vi "Write_output_file.vi"(0 "Output filename":path, 1 "Header":string, 2 "Template Filename":path, 5 "Channel Names":string[](array[string]), 7 "Data":string[][](array[string]), 9 "Desired Columns":i32[](array[numeric])=[0, 1, 2, 3, 4, 5, 6, 7, 8, 9, 10, 11, 12, 13, 14, 15, 16, 17, 18, 19, 20, 21, 22, 23, 24, 25, 26, 27, 28, 29, 30, 31, 32, 33, 34, 35, 36, 37, 38, 39, 40, 41, 42, 43, 44, 45, 46, 47, 48, 49, 50, 51, 52, 53, 54, 55, 56, 57, 58, 59, 60, 61, 62, 63, 64, 65, 66, 67, 68, 69, 70, 71, 72, 73, 74, 75, 76, 77, 78, 79, 80, 81, 82, 83, 84, 85, 86, 87, 88, 89, 90, 91, 92, 93, 94, 95, 96, 97, 98, 99, 100, 101, 102, 103, 104, 105, 106, 107, 108, 109, 110, 111, 112, 113, 114, 115, 116, 117, 118, 119, 120, 121, 122, 123, 124, 125, 126, 127, 128, 129, 130, 131, 132, 133, 134, 135, 136, 137, 138, 139, 140, 141, 142, 143, 144, 145, 146, 147, 148, 149, 150, 151, 152, 153, 154, 155, 156, 157, 158, 159, 160, 161, 162, 163, 164, 165, 166, 167, 168, 169, 170, 171, 172, 173, 174, 175, 176, 177, 178, 179, 180, 181, 182, 183, 184, 185, 186, 187, 188, 189, 190, 191, 192, 193, 194, 195, 196, 197, 198, 199, 200, 201, 202, 203, 204, 205, 206, 207, 208, 209, 210, 211, 212, 213, 214, 215, 216, 217, 218, 219, 220, 221, 222, 223, 224, 225, 226, 227, 228, 229, 230, 231, 232, 233, 234], 11 "Simple Save?":bool, 12 "Save Plotted rows only?":bool, 13 "Summarise mode":T2(ring), 14 "Grouping info":T3[](array[typedef]), 15 "Channels to Tabulate in header":i32[](listbox)) -> (4 "Output filename Out":path)   [LabVIEW 2020]
uses:
  Controls/Group_Binning.ctl
  Results_plotter_Global.vi
panel:
  out "Which Button?":T1(ring)=enum."Center Button"
  out "Table Values":string[][](array[string])
  out "Table Names":string[](array[string])
  out "Table":string
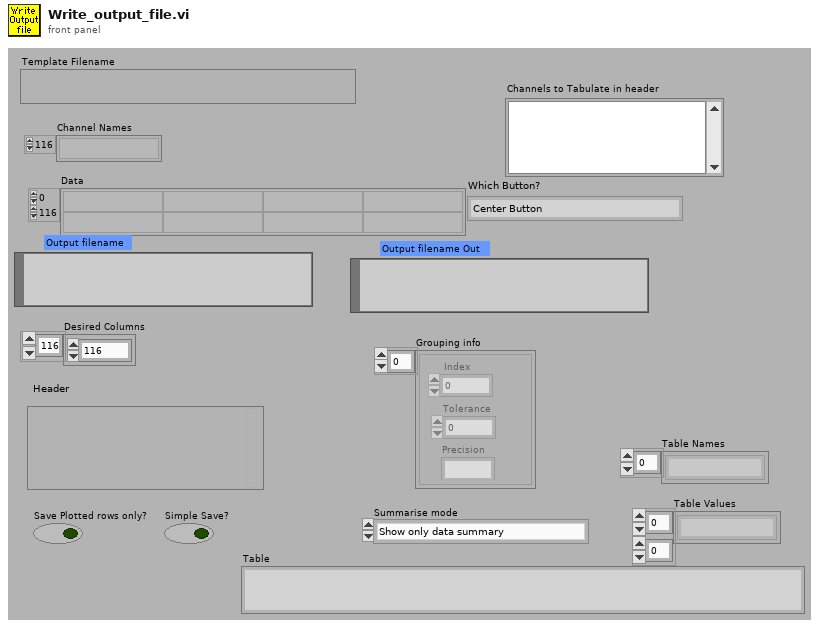
[diagram p1: front panel]
types:
  T1 = enum16{"Left Button", "Center Button", "Right Button", "Window Close"}
  T2 = enum16{"Show only data summary", "Show data summary", "No data summary"}
  T3 = typedef "Group_Binning.ctl" = cluster{"Index":i32, "Tolerance":dbl, "Precision":string}
  T4 = typedef "Dispose_Channel.ctl" = enum16{"Always", "If Blank", "Never"}
  T5 = enum32{"existing file", "new file", "new or existing file", "existing dir", "new dir", "new or existing dir", "existing file (use LLBs)", "new file (use LLBs)", "new or existing file (use LLBs)", "new or existing file or directory (use LLBs)"}
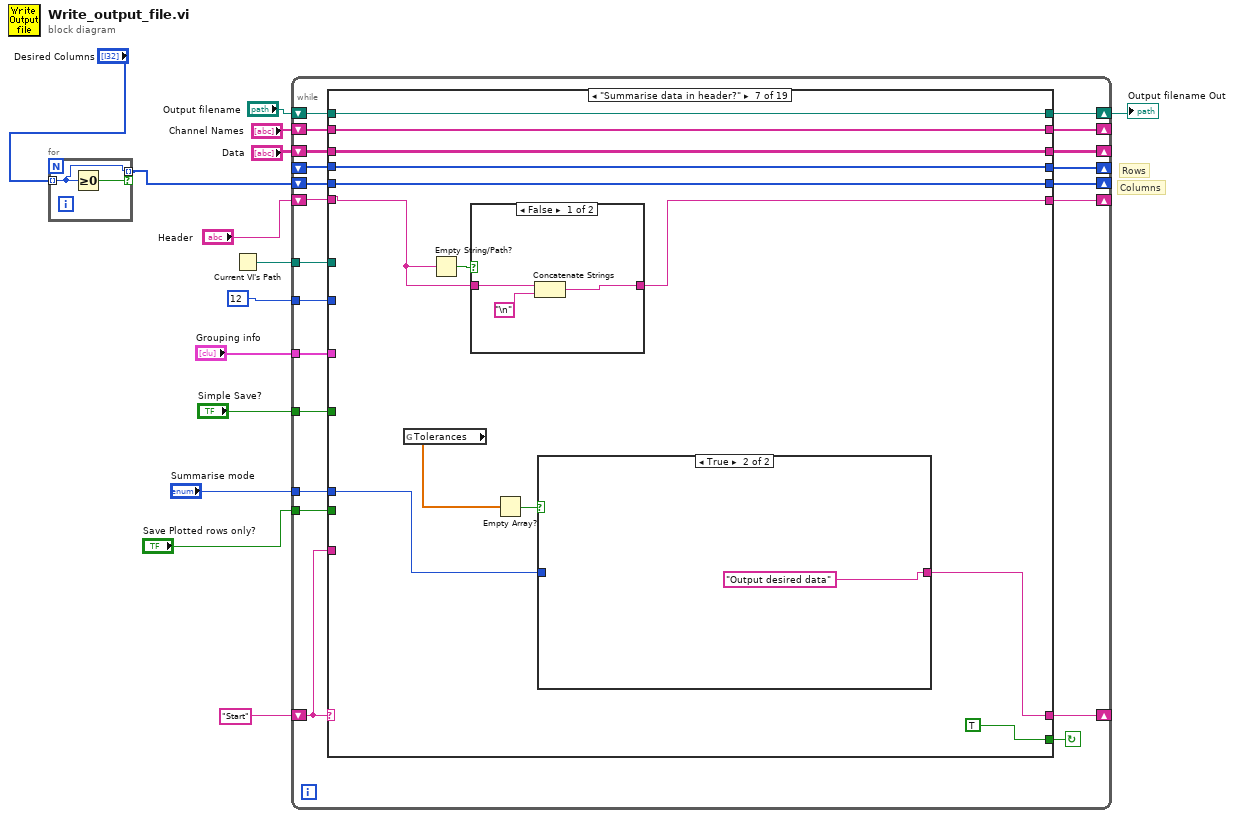
[diagram p0: block diagram]
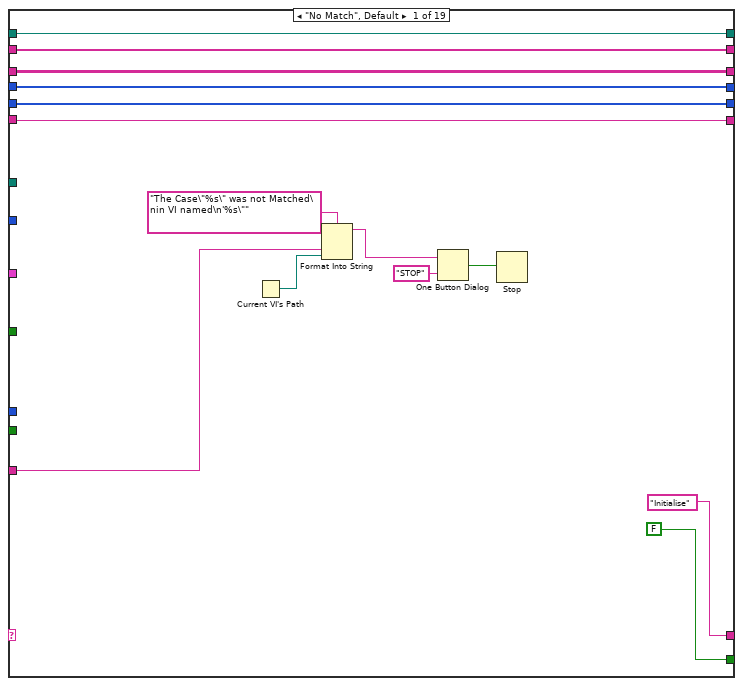
[diagram p2: hidden frame]
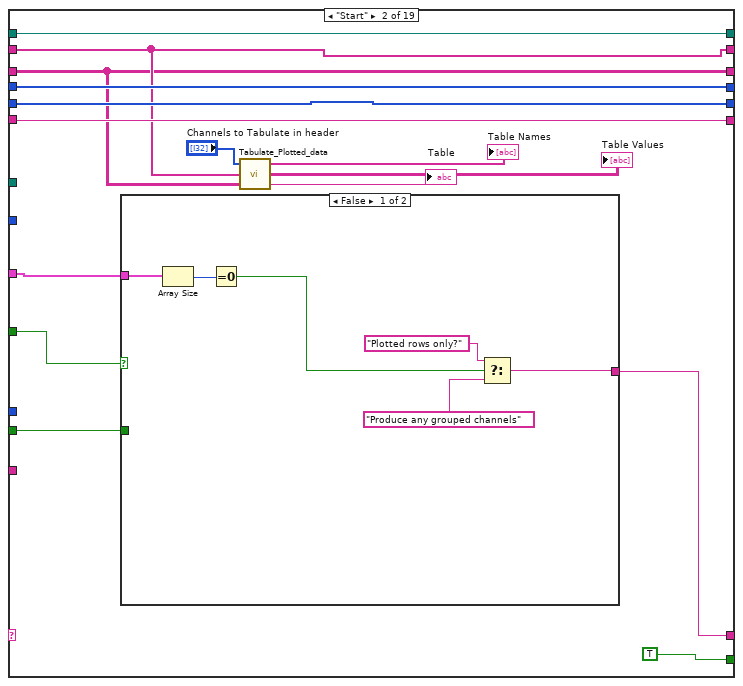
[diagram p3: hidden frame]
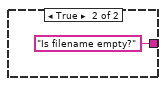
[diagram p4: hidden frame]
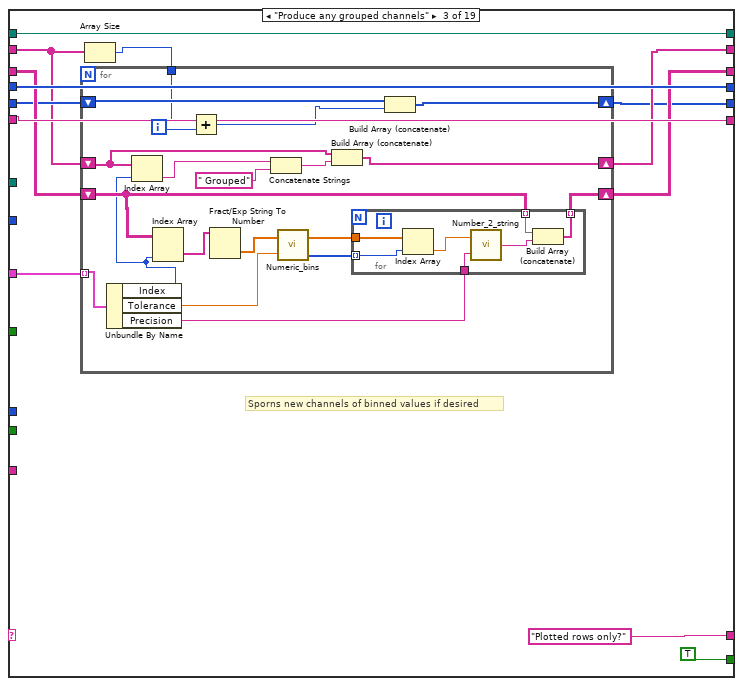
[diagram p5: hidden frame]
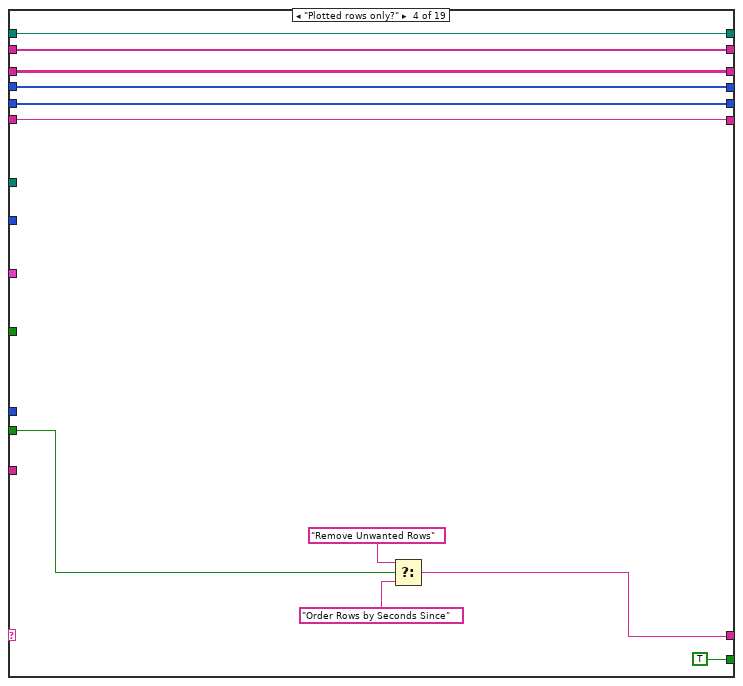
[diagram p6: hidden frame]
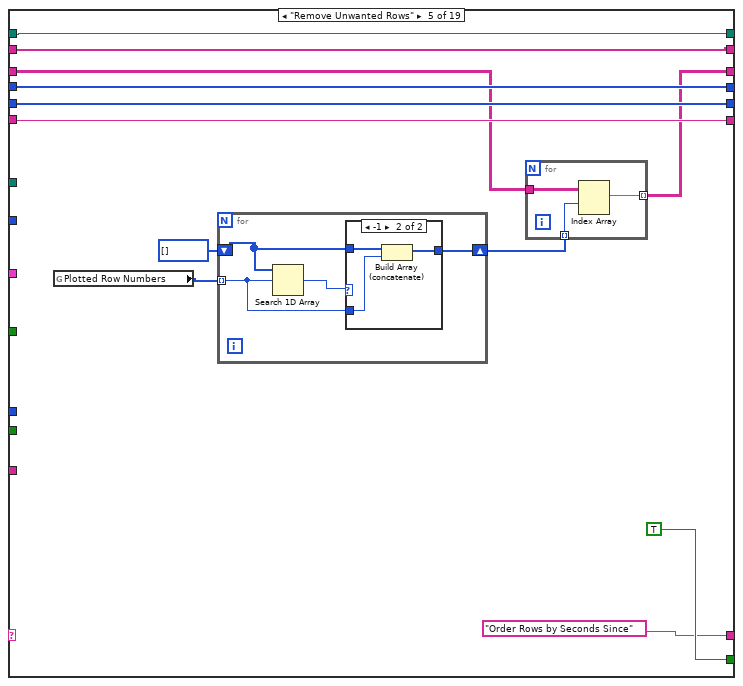
[diagram p7: hidden frame]
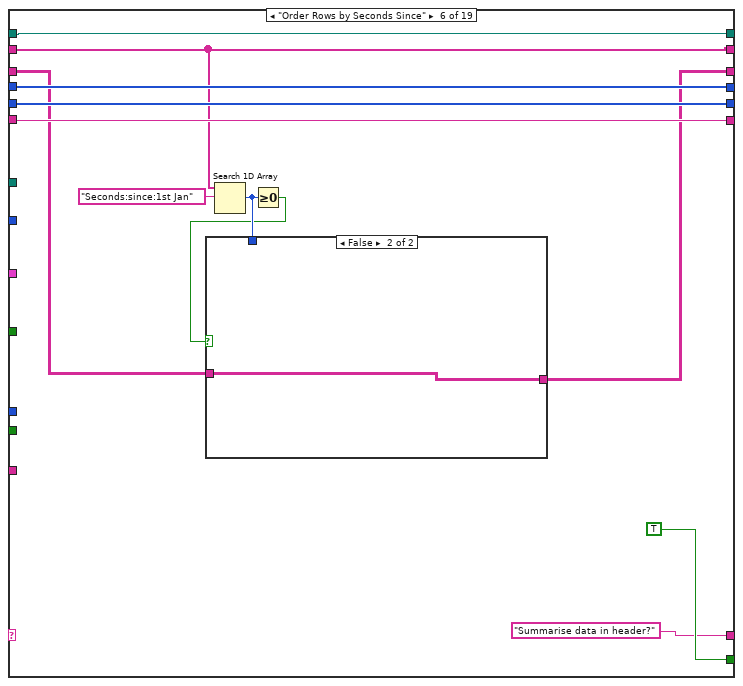
[diagram p9: hidden frame]
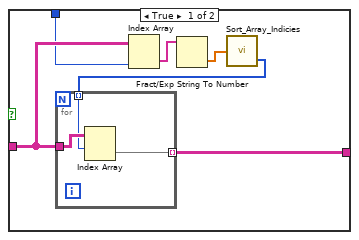
[diagram p10: hidden frame]
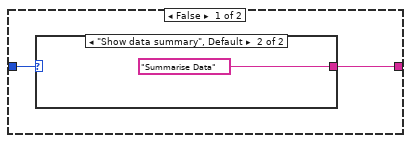
[diagram p11: hidden frame]
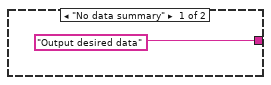
[diagram p12: hidden frame]
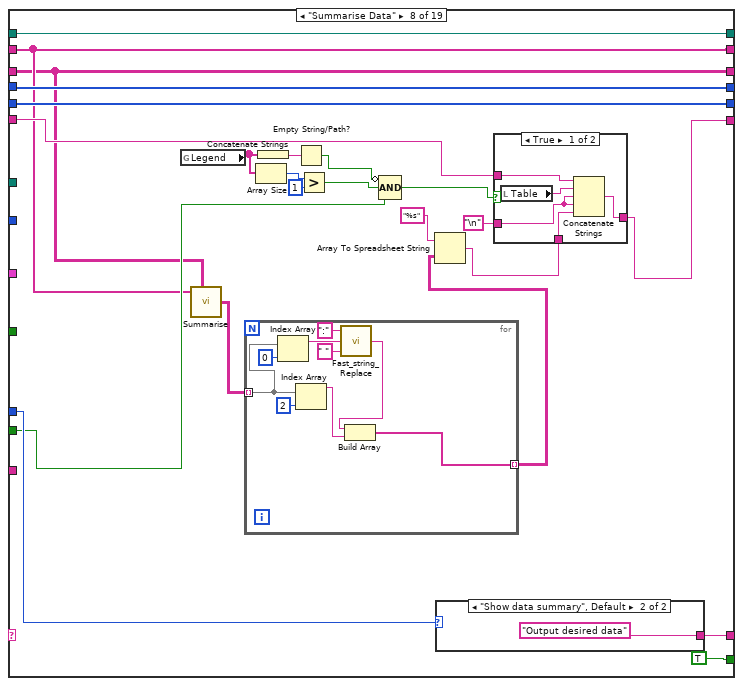
[diagram p14: hidden frame]
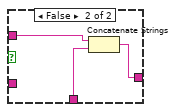
[diagram p15: hidden frame]
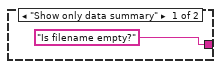
[diagram p16: hidden frame]
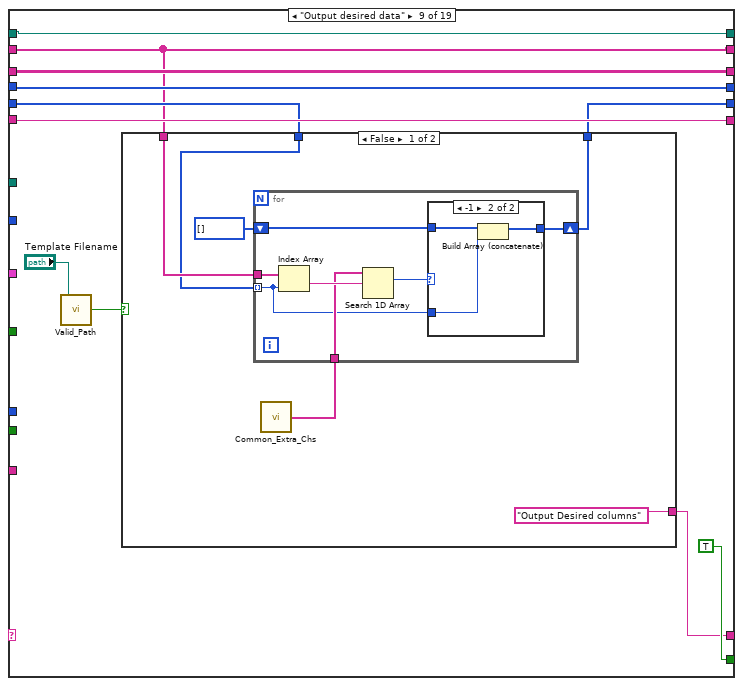
[diagram p17: hidden frame]
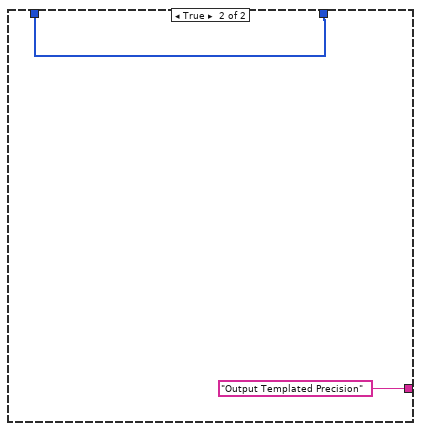
[diagram p19: hidden frame]
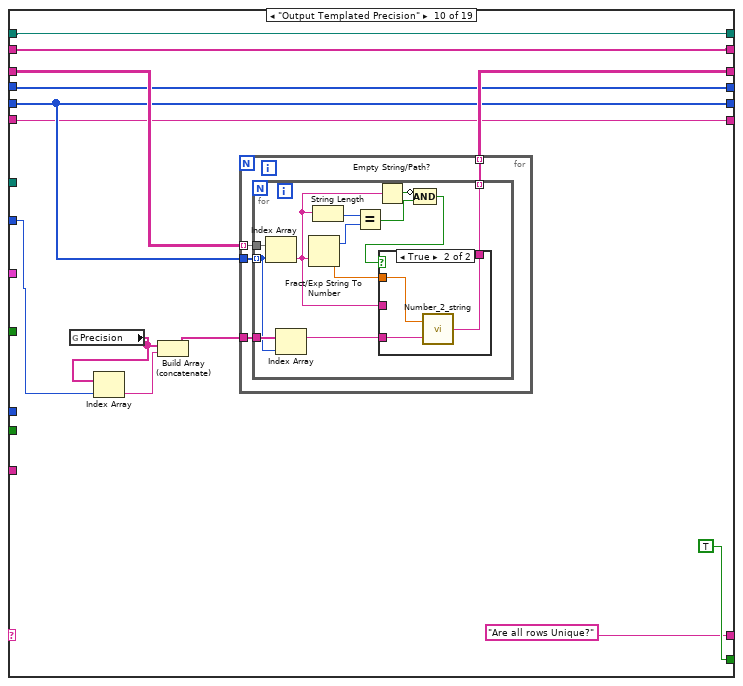
[diagram p20: hidden frame]
diagram:
  # "Columns"
  # "Rows"
  n1 = for {
    tunnel: "Desired Columns" -> [w16] mode=indexing
    tunnel: [w16] -> w1 mode=indexing if=w15
    n2 = Greater Or Equal To 0?(x=w16) -> (x >= 0?=w15:bool)
  }
  n3 = Current VI's Path() -> (path=w12:path)
  n4 = while {
    shift-left: "Header" -> [w27]
    shift-right: [w30] -> _
    shift-left: w1 -> [w29]
    shift-right: [w28] -> _
    shift-left: _ -> [w31]
    shift-right: [w32] -> _
    shift-left: "Data" -> [w34]
    shift-right: [w33] -> _
    shift-left: "Start" -> [w35]
    shift-right: [w36] -> _
    tunnel: w12 -> [w26]
    shift-right: [w25] -> w11
    shift-left: "Output filename" -> [w24]
    shift-right: [w22] -> _
    shift-left: "Channel Names" -> [w23]
    tunnel: "Simple Save?" -> [w21]
    tunnel: 12 ("disabled index (col)") -> [w20]
    tunnel: "Grouping info" -> [w19]
    tunnel: "Summarise mode" -> [w18]
    tunnel: "Save Plotted rows only?" -> [w17]
    stop <- w37 continue-if-true
    n5 = case shown="\"Summarise data in header?\"" w35 {
      tunnel: [FALSE TRUE TRUE TRUE ("cancelled") TRUE TRUE TRUE TRUE TRUE TRUE TRUE TRUE TRUE TRUE w401 w418 TRUE ("cancelled") FALSE ("cancelled") FALSE] -> w37
      tunnel: ["Initialise" w63 "Plotted rows only?" w115 "Order Rows by Seconds Since" "Summarise data in header?" w180 w210 w241 "Are all rows Unique?" "Is filename empty?" w317 "Remove Blank Columns" "Is filename empty?" w402 w419 "Write File" "End" "End"] -> w36
      tunnel: w35 -> [w46 _ _ _ _ _ _ _ _ _ _ _ _ _ _ _ _ _ _]
      tunnel: w34 -> [w43 w56 w82 w119 w131 w150 w176 w193 w238 w275 w304 w324 w360 w365 w406 w428 w448 w463 w489]
      tunnel: [w43 w56 w80 w119 w130 w149 w176 w193 w238 w274 w299 w324 w359 w369 w406 w428 w448 w463 w489] -> w33
      tunnel: [w42 w65 w85 w118 w135 w158 w181 w213 w243 w273 w303 w323 w358 w375 w407 w429 w451 w472 w496] -> w32
      tunnel: w31 -> [w42 w65 w85 w118 w135 w158 w181 w213 w243 w273 w303 _ w358 w375 w407 w429 w451 w472 w496]
      tunnel: [w40 w64 w83 w116 w134 w157 w172 w211 w242 w271 w301 w315 w355 w373 w408 w430 w443 w473 w488] -> w30
      tunnel: w29 -> [w41 w60 w78 w117 w133 w156 w175 w212 w240 w272 w302 w316 w356 w371 w409 w431 w446 w454 w495]
      tunnel: [w41 w60 w75 w117 w133 w156 w175 w212 w239 w272 w302 w316 w356 w367 w409 w431 w446 w454 w495] -> w28
      tunnel: w27 -> [w40 w64 w83 w116 w134 w157 w173 w195 w242 w271 w301 w315 w355 w373 w408 w430 w441 w473 w488]
      tunnel: w26 -> [_ _ _ _ _ _ _ _ _ _ _ _ _ _ _ _ _ _ _]
      tunnel: [w39 w62 w84 w121 w127 w154 w179 w209 w237 w269 w298 w314 w354 w372 w405 w417 w445 w459 w491] -> w25
      tunnel: w24 -> [w39 w62 w84 w121 w127 w154 w179 w209 w237 w269 w298 w314 w354 w372 w398 w417 w445 w459 w491]
      tunnel: w23 -> [w38 w57 w77 w120 w126 w148 w177 w194 w236 w268 w297 w313 w353 w366 w400 w426 w447 w456 w492]
      tunnel: [w38 w57 w79 w120 w126 w148 w177 w194 w236 w268 w297 w313 w353 w366 w400 w426 w447 w456 w492] -> w22
      tunnel: w21 -> [_ w61 _ _ _ _ _ _ _ _ _ _ _ _ _ _ _ w455 w490]
      tunnel: w20 -> [_ _ _ _ _ _ _ _ _ w267 _ _ _ _ _ _ _ _ _]
      tunnel: w19 -> [_ w54 w81 _ _ _ _ _ _ _ _ _ _ _ _ _ _ _ _]
      tunnel: w18 -> [_ _ _ _ _ _ w178 w208 _ _ _ _ _ _ _ _ _ _ w487]
      tunnel: w17 -> [_ w59 _ w123 _ _ _ w207 _ _ _ _ _ _ _ _ _ _ _]
      frame "No Match", Default {
        n6 = Current VI's Path() -> (path=w45:path)
        n7 = Format Into String(format string="The Case\"%s\" was not Matched\nin VI named\n'%s\"" ("Format String"), w46, w45) -> (resulting string=w49:string)  [unwired: 2 in, 1 out]
        n8 = One Button Dialog(message=w49, button name ("OK")="STOP") -> (true=w47:bool)
        n9 = Stop(stop? (T)=w47) -> ()
      }
      frame "Start" {
        n10 = case shown="False" w61 {
          tunnel: [w67 "Is filename empty?" ("f")] -> w63
          tunnel: w59 -> [_ _]
          tunnel: w54 -> [w71 _]
          frame False {
            n11 = Array Size(array=w71) -> (size(s)=w72:i32)
            n12 = Equal To 0?(x=w72) -> (x = 0?=w70:bool)
            n13 = Select(t="Plotted rows only?", s=w70, f="Produce any grouped channels") -> (s? t:f=w67:string)
          }
          frame True {
          }
        }
        n14 = call "Tabulate_Plotted_data.vi"("Data"=w56, "Channel Names"=w57, "Channels to Tabulate"="Channels to Tabulate in header") -> ("spreadsheet string"=→"Table":string, "Channel Values"=→"Table Values":string[][], "Channel Names"=→"Table Names":string[])
      }
      frame "Produce any grouped channels" {
        # "Sporns new channels of binned values if desired"
        n15 = Array Size(array=w77) -> (size(s)=w76:i32)
        n16 = for {
          shift-right: [w98] -> w80
          shift-left: w82 -> [w99]
          tunnel: w81 -> [w103] mode=indexing
          shift-right: [w92] -> w79
          shift-left: w77 -> [w93]
          shift-right: [w90] -> w75
          shift-left: w78 -> [w91]
          tunnel: w76 -> [w88]
          i -> [w89]
          n17 = Unbundle By Name(w103) -> ("Index"=w97:i32, "Tolerance"=w101:dbl, "Precision"=w100:string)
          n18 = Index Array(array=w93, index=w97) -> (element=w95:string)
          n19 = Index Array(array=w99, index (col)=w97) -> (element=w102:string[])  [unwired: 1 in]
          n20 = Add(x=w88, y=w89) -> (x+y=w87:i32)
          n21 = Fract/Exp String To Number(string=w102) -> (number=w106:dbl[])  [unwired: 4 out]
          n22 = Concatenate Strings(w95, " Grouped" ("string")) -> (w94:string)
          n23 = call "Numeric_bins.vi"("Values"=w106, "Tolerance"=w101) -> ("Bin Centres"=w105:dbl[], "Bin Index"=w104:i32[])  [unwired: 1 out]
          n24 = Build Array (concatenate)(w93, w94) -> (w92:string[])
          n25 = for {
            tunnel: w105 -> [w113]
            tunnel: w104 -> [w112] mode=indexing
            tunnel: [w109] -> w98 mode=indexing
            tunnel: w100 -> [w108]
            tunnel: w99 -> [w107] mode=indexing
            n26 = Index Array(array=w113, index=w112) -> (element=w111:dbl)
            n27 = call "Number_2_string.vi"("precision"=w108, "number"=w111) -> ("String"=w110:string)
            n28 = Build Array (concatenate)(w107, w110) -> (w109:string[])
          }
          n29 = Build Array (concatenate)(w91, w87) -> (w90:i32[])
        }
      }
      frame "Plotted rows only?" {
        n30 = Select(t="Remove Unwanted Rows" ("f"), s=w123, f="Order Rows by Seconds Since") -> (s? t:f=w115:string)
      }
      frame "Remove Unwanted Rows" {
        n31 = global read "Results_plotter_Global.vi" "Plotted Row Numbers"() -> (w125:i32[])
        n32 = for {
          shift-right: [w141] -> w129
          shift-left: i32[] [] -> [w142]
          tunnel: w125 -> [w140] mode=indexing
          n33 = Search 1D Array(1D array=w142, element=w140) -> (index of element=w143:i32)  [unwired: 1 out]
          n34 = case shown="-1" w143 {
            tunnel: w142 -> [w144 w147]
            tunnel: [w144 w146] -> w141
            tunnel: w140 -> [_ w145]
            frame 0, Default {
            }
            frame -1 {
              n35 = Build Array (concatenate)(w147, w145) -> (w146:i32[])
            }
          }
        }
        n36 = for {
          tunnel: w129 -> [w139] mode=indexing
          tunnel: w131 -> [w138]
          tunnel: [w137] -> w130 mode=indexing
          n37 = Index Array(array=w138, index (row)=w139) -> (element=w137:string[])  [unwired: 1 in]
        }
      }
      frame "Order Rows by Seconds Since" {
        n38 = Search 1D Array(1D array=w148, element="Seconds:since:1st Jan" ("Ch Name out")) -> (index of element=w152:i32)  [unwired: 1 in]
        n39 = Greater Or Equal To 0?(x=w152) -> (x >= 0?=w151:bool)
        n40 = case shown="False" w151 {
          tunnel: [w165 w169] -> w149
          tunnel: w150 -> [w164 w169]
          tunnel: w152 -> [w163 _]
          frame True {
            n41 = Index Array(array=w164, index (col)=w163) -> (element=w162:string[])  [unwired: 1 in]
            n42 = Fract/Exp String To Number(string=w162) -> (number=w161:dbl[])  [unwired: 3 in, 1 out]
            n43 = call "Sort_Array_Indicies.vi"("unsorted array"=w161) -> ("Sort Index"=w160:i32[])  [unwired: 1 out]
            n44 = for {
              tunnel: w164 -> [w168]
              tunnel: [w166] -> w165 mode=indexing
              tunnel: w160 -> [w167] mode=indexing
              n45 = Index Array(array=w168, index (row)=w167) -> (element=w166:string[])  [unwired: 1 in]
            }
          }
          frame False {
          }
        }
      }
      frame "Summarise data in header?" {
        n46 = global read "Results_plotter_Global.vi" "Tolerances"() -> (w170:dbl[])
        n47 = Empty String/Path?(string/path=w173) -> (empty?=w174:bool)
        n48 = case shown="False" w174 {
          tunnel: [w188 w191] -> w172
          tunnel: w173 -> [w189 w191]
          frame False {
            n49 = Concatenate Strings(w189, "\n") -> (w188:string)
          }
          frame True {
          }
        }
        n50 = Empty Array?(array=w170) -> (empty?=w171:bool)
        n51 = case shown="True" w171 {
          tunnel: [w184 "Output desired data" ("t")] -> w180
          tunnel: w178 -> [w183 _]
          frame False {
            n52 = case shown="\"Show data summary\", Default" w183 {
              tunnel: ["Output desired data" ("t") "Summarise Data"] -> w184
              frame "No data summary" {
              }
              frame "Show data summary", Default {
              }
            }
          }
          frame True {
          }
        }
      }
      frame "Summarise Data" {
        n53 = global read "Results_plotter_Global.vi" "Legend"() -> (w200:string[])
        n54 = call "Summarise.vi"("Channel Names"=w194, "Data"=w193) -> ("Summary"=w205:string[][])  [unwired: 2 in, 1 out]
        n55 = for {
          tunnel: w205 -> [w229] mode=indexing
          tunnel: [w223] -> w192 mode=indexing
          n56 = Index Array(array=w229, index=0) -> (element=w227:string)
          n57 = Index Array(array=w229, index=2) -> (element=w228:string)
          n58 = call "Fast_string_Replace.vi"("Replace match with:"=" ", "Input String"=w227, "regular expression"=":") -> ("Output String"=w224:string)  [unwired: 2 out]
          n59 = Build Array(w224, w228) -> (w223:string[])
        }
        n60 = Array Size(array=w200) -> (size(s)=w199:i32)
        n61 = Concatenate Strings(w200) -> (w202:string)
        n62 = Empty String/Path?(string/path=w202) -> (empty?=w197:bool)
        n63 = Greater?(x=w199, y=1) -> (0:w196:bool)
        n64 = Compound Arithmetic op=AND(invert w197, w196, w207) -> (w201:bool)
        n65 = Array To Spreadsheet String(array=w192, 3:"%s" ("format string")) -> (spreadsheet string=w204:string)  [unwired: 1 out]
        n66 = case shown="\"Show data summary\", Default" w208 {
          tunnel: ["Is filename empty?" "Output desired data"] -> w210
          frame "Show only data summary" {
          }
          frame "Show data summary", Default {
          }
        }
        n67 = case shown="True" w201 {
          tunnel: [w216 w221] -> w211
          tunnel: w195 -> [w219 w220]
          tunnel: w204 -> [w217 w222]
          tunnel: "\n" -> [w218 _]
          frame True {
            n68 = local read "Table"() -> (w215:string)
            n69 = Concatenate Strings(w219, w215, w218, w218, w217) -> (w216:string)
          }
          frame False {
            n70 = Concatenate Strings(w220, w222) -> (w221:string)
          }
        }
      }
      frame "Output desired data" {
        n71 = call "Valid_Path.vi"("Filename"="Template Filename") -> ("Valid Path?"=w234:bool)
        n72 = case shown="False" w234 {
          tunnel: ["Output Desired columns" "Output Templated Precision" ("f")] -> w241
          tunnel: w240 -> [w248 w262]
          tunnel: [w246 w262] -> w239
          tunnel: w236 -> [w249 _]
          frame False {
            n73 = call "Common_Extra_Chs.vi"() -> ("Common Extra Channels"=w245:string[])
            n74 = for {
              shift-right: [w251] -> w246
              shift-left: i32[] [] -> [w253]
              tunnel: w249 -> [w257]
              tunnel: w248 -> [w252] mode=indexing
              tunnel: w245 -> [w255]
              n75 = Index Array(array=w257, index=w252) -> (element=w256:string)
              n76 = Search 1D Array(1D array=w255, element=w256) -> (index of element=w254:i32)  [unwired: 1 out]
              n77 = case shown="-1" w254 {
                tunnel: w253 -> [w258 w261]
                tunnel: w252 -> [_ w260]
                tunnel: [w258 w259] -> w251
                frame 0, Default {
                }
                frame -1 {
                  n78 = Build Array (concatenate)(w261, w260) -> (w259:i32[])
                }
              }
            }
          }
          frame True {
          }
        }
      }
      frame "Output Templated Precision" {
        n79 = global read "Results_plotter_Global.vi" "Precision"() -> (w266:string[])
        n80 = Index Array(array=w266, index=w267) -> (element=w264:string)
        n81 = Build Array (concatenate)(w266, w264) -> (w265:string[])
        n82 = for {
          tunnel: w272 -> [w280]
          tunnel: w275 -> [w279] mode=indexing
          tunnel: w265 -> [w278]
          tunnel: [w277] -> w274 mode=indexing
          n83 = for {
            tunnel: w280 -> [w290] mode=indexing
            tunnel: w279 -> [w292]
            tunnel: w278 -> [w291]
            tunnel: [w284] -> w277 mode=indexing
            n84 = Index Array(array=w292, index=w290) -> (element=w283:string)
            n85 = Index Array(array=w291, index=w290) -> (element=w282:string)
            n86 = Fract/Exp String To Number(string=w283) -> (offset past number=w288:i32, number=w285:dbl)  [unwired: 3 out]
            n87 = String Length(string=w283) -> (length=w289:i32)
            n88 = Equal?(x=w289, y=w288) -> (x = y?=w286:bool)
            n89 = Empty String/Path?(string/path=w283) -> (empty?=w287:bool)
            n90 = Compound Arithmetic op=AND(invert w287, w286) -> (w281:bool)
            n91 = case shown="True" w281 {
              tunnel: w282 -> [_ w295]
              tunnel: w285 -> [_ w296]
              tunnel: [w293 w294] -> w284
              tunnel: w283 -> [w293 _]
              frame False {
              }
              frame True {
                n92 = call "Number_2_string.vi"("precision"=w295, "number"=w296) -> ("String"=w294:string)
              }
            }
          }
        }
      }
      frame "Output Desired columns" {
        n93 = for {
          tunnel: w302 -> [w308]
          tunnel: w304 -> [w307] mode=indexing
          tunnel: [w306] -> w299 mode=indexing
          n94 = for {
            tunnel: w308 -> [w310] mode=indexing
            tunnel: w307 -> [w311]
            tunnel: [w309] -> w306 mode=indexing
            n95 = Index Array(array=w311, index=w310) -> (element=w309:string)
          }
        }
      }
      frame "Are all rows Unique?" {
        n96 = for {
          shift-right: [w330] -> _
          shift-left: _ -> [w329]
          tunnel: w324 -> [w332] mode=indexing
          shift-right: [w328] -> w323
          shift-left: _ -> [w327]
          tunnel: [w326] -> w320
          i -> [w326]
          n97 = Array To Spreadsheet String(array=w332, 3:"%s" ("format string")) -> (spreadsheet string=w331:string)  [unwired: 1 out]
          n98 = case shown="1, Default" w326 {
            tunnel: w331 -> [w337 w343]
            tunnel: [w336 w340] -> w330
            tunnel: w329 -> [_ w344]
            tunnel: [w334 w341] -> w328
            tunnel: w327 -> [_ w342]
            tunnel: w326 -> [_ w338]
            frame 0 {
              n99 = Build Array(w337) -> (w336:string[])
              n100 = Build Array(0) -> (w334:i32[])
            }
            frame 1, Default {
              n101 = Search 1D Array(1D array=w344, element=w343) -> (index of element=w339:i32)  [unwired: 1 out]
              n102 = case shown="-1" w339 {
                tunnel: w344 -> [w346 w352]
                tunnel: w343 -> [_ w351]
                tunnel: w342 -> [w345 w350]
                tunnel: [w345 w349] -> w341
                tunnel: [w346 w348] -> w340
                tunnel: w338 -> [_ w347]
                frame 0, Default {
                }
                frame -1 {
                  n103 = Build Array (concatenate)(w352, w351) -> (w348:string[])
                  n104 = Build Array (concatenate)(w350, w347) -> (w349:i32[])
                }
              }
            }
          }
        }
        n105 = Array Size(array=w323) -> (size(s)=w322:i32)
        n106 = Decrement(x=w322) -> (x-1=w321:i32)
        n107 = Equal?(x=w321, y=w320) -> (x = y?=w312:bool)
        n108 = Select(t="Remove Blank Columns", s=w312, f="Remove Duplicate Rows") -> (s? t:f=w317:string)
      }
      frame "Remove Duplicate Rows" {
        n109 = for {
          tunnel: w358 -> [w364] mode=indexing
          tunnel: w360 -> [w363]
          tunnel: [w362] -> w359 mode=indexing
          n110 = Index Array(array=w363, index (row)=w364) -> (element=w362:string[])  [unwired: 1 in]
        }
      }
      frame "Remove Blank Columns" {
        n111 = global read "Results_plotter_Global.vi" "Dispose"() -> (w370:T4[])
        n112 = for {
          tunnel: w371 -> [w384] mode=indexing
          tunnel: w370 -> [w388]
          tunnel: w365 -> [w386]
          tunnel: [w385] -> w368 mode=indexing if=w383
          tunnel: [w384] -> w367 mode=indexing if=w383
          i -> [w385]
          n113 = Index Array(array=w388, index=w384) -> (element=w387:T4)
          n114 = case shown="\"If Blank\"" w387 {
            tunnel: w386 -> [_ w395]
            tunnel: w385 -> [_ w394]
            tunnel: [TRUE w390] -> w383
            frame Default {
            }
            frame "If Blank" {
              n115 = Index Array(array=w395, index (col)=w394) -> (element=w393:string[])  [unwired: 1 in]
              n116 = Concatenate Strings(w393) -> (w392:string)
              n117 = Empty String/Path?(string/path=w392) -> (empty?=w391:bool)
              n118 = Not(x=w391) -> (.not. x?=w390:bool)
            }
          }
        }
        n119 = for {
          tunnel: w368 -> [w379]
          tunnel: w365 -> [w378] mode=indexing
          tunnel: [w377] -> w369 mode=indexing
          n120 = for {
            tunnel: w379 -> [w382] mode=indexing
            tunnel: w378 -> [w381]
            tunnel: [w380] -> w377 mode=indexing
            n121 = Index Array(array=w381, index=w382) -> (element=w380:string)
          }
        }
      }
      frame "Is filename empty?" {
        n122 = call "Append_Suffiix.vi"("Results file"=w398) -> ("appended path"=w397:path)
        n123 = call "Valid_Path.vi"("Filename"=w397) -> ("Valid Path?"=w399:bool)
        n124 = case shown="False" w399 {
          tunnel: [w410 w416] -> w405
          tunnel: w397 -> [_ w416]
          tunnel: [w412 TRUE ("cancelled")] -> w401
          frame False {
            (unwired) T5."new or existing file" ("select mode (2)")
            n125 = File Dialog(7:"Save Output file as:" ("prompt")) -> (1:w413:bool, 3:w411:path)  [unwired: 1 in, 7 out]
            n126 = Not(x=w413) -> (.not. x?=w412:bool)
            n127 = call "Append_Suffiix.vi"("Results file"=w411) -> ("appended path"=w410:path)
          }
          frame True {
          }
        }
        n128 = call "Does_file_exist_(simple).vi"("Pathname"=w405) -> ("exists?"=w404:bool)
        n129 = Select(t="Check for overwrite or append", s=w404, f="Write File") -> (s? t:f=w402:string)
      }
      frame "Check for overwrite or append" {
        n130 = Format Into String(format string="Do you want to append to the result file\n\"%s\"" ("message"), w417) -> (resulting string=w424:string)  [unwired: 2 in, 1 out]
        n131 = call <vilib>:"Three Button Dialog.vi"("Window Title (\"\")"="Output File Dialog" ("Window Title (\"\")"), "Right Button Text (\"Cancel\")"="Cancel" ("Button 3 Name"), "Center Button Text (\"No\")"="Overwrite" ("F button name (\"Cancel\")"), "Left Button Text (\"Yes\")"="Append" ("T button name (\"OK\")"), "message"=w424) -> ("Which Button?"=w425:T1)  [unwired: 6 out]
        "Which Button?" <- w425
        n132 = case shown="\"Center Button\"" w425 {
          tunnel: ["Append and Merge Results file" ("t") "Write File" "End" ("t") "End"] -> w419
          tunnel: [TRUE TRUE FALSE FALSE] -> w418
          tunnel: w417 -> [_ w434 _ _]
          frame "Left Button" {
          }
          frame "Center Button" {
            n133 = Delete(path (use dialog)=w434) -> ()  [unwired: 4 in, 3 out]
          }
          frame "Right Button" {
          }
          frame "Window Close" {
          }
        }
      }
      frame "Append to Results file" {
        w442 = "\n"
        n134 = call "Read_File_Simple.vi"("Filename"=w445) -> ("string"=w444:string)  [unwired: 2 in, 7 out]
        n135 = Concatenate Strings(w444, w442, w442, w442, w441) -> (w443:string)
      }
      frame "Append and Merge Results file" {
        w452 = FALSE  # Delete First Rows?
        w460 = TRUE  # Read Channel Names only
        w462 = FALSE  # Append last row only
        w466 = TRUE  # exists?
        w469 = FALSE  # Present Channels only
        n136 = case shown="False" w455 {
          tunnel: w454 -> [w476 _]
          tunnel: w456 -> [w475 w480]
          tunnel: [w474 w480] -> w453
          frame False {
            n137 = for {
              tunnel: w476 -> [w477] mode=indexing
              tunnel: w475 -> [w479]
              tunnel: [w478] -> w474 mode=indexing
              n138 = Index Array(array=w479, index=w477) -> (element=w478:string)
            }
          }
          frame True {
          }
        }
        n139 = call "Read_Data_file.vi"("Results file"=w459, "Read Channel Names only"=w460, "Delete First Rows?"=w452, "Template File"=path "") -> ("String Before"=w458:string)  [unwired: 3 in, 12 out]
        n140 = String Length(string=w458) -> (length=w457:i32)
        n141 = call "Check_and_rewrite_file.vi"("Filename"=w459, "Present Channels only"=w469, "Present Channels"=w453, "Start of read offset (chars.: 0)"=w457) -> ("Merged Channels"=w468:string[], "Merged?"=w467:bool)  [unwired: 10 out]
        n142 = case shown="True" w467 {
          tunnel: [w482 w484] -> w465
          tunnel: w453 -> [w482 w486]
          tunnel: w463 -> [w481 w485]
          tunnel: [w481 w483] -> w464
          tunnel: w468 -> [_ w484]
          frame False {
          }
          frame True {
            n143 = call "Merge_2D_values.vi"("Values In"=w485, "Present Channels"=w486, "Desired Channels"=w484) -> ("Values Out"=w483:string[][])
          }
        }
        n144 = call "Write_Ch_data_file.vi"("Append last row only"=w462, "Header string"=w458, "exists?"=w466, "Channel Values"=w464, "Channel names"=w465, "Filename"=w459) -> ()  [unwired: 1 in, 5 out]
      }
      frame "Write File" {
        n145 = case shown="\"Show data summary\", Default" w487 {
          tunnel: w495 -> [_ w523]
          tunnel: w492 -> [_ w522]
          tunnel: w491 -> [w502 w520]
          tunnel: w490 -> [_ w517]
          tunnel: w489 -> [_ w515]
          tunnel: w488 -> [_ w513]
          frame "Show only data summary" {
            w503 = FALSE  # Present Channels only
            n146 = local read "Table Values"() -> (w498:string[][])
            n147 = local read "Table Names"() -> (w501:string[])
            n148 = local read "Which Button?"() -> (w500:T1)
            n149 = call "Check_and_rewrite_file.vi"("Filename"=w502, "Present Channels only"=w503, "Present Channels"=w501) -> ("Merged Channels"=w504:string[])  [unwired: 1 in, 11 out]
            n150 = for {
              tunnel: w498 -> [w506] mode=indexing
              tunnel: [w505] -> w497 mode=indexing
              n151 = for {
                tunnel: w506 -> [w508] mode=indexing
                tunnel: [w507] -> w505 mode=indexing
                n152 = call "Truncate_Excessive_Strings.vi"("String"=w508) -> ("Truncated String"=w507:string)  [unwired: 2 in]
              }
            }
            n153 = case shown="\"Center Button\"" w500 {
              tunnel: [w509 FALSE ("exists?")] -> w499
              frame "Left Button", Default {
                w509 = TRUE  # exists?
              }
              frame "Center Button" {
              }
            }
            n154 = call "Write_Ch_data_file.vi"("exists?"=w499, "Channel Values"=w497, "Channel names"=w504, "Filename"=w502) -> ()  [unwired: 4 in, 4 out]
          }
          frame "Show data summary", Default {
            w519 = FALSE  # Append last row only
            w521 = FALSE  # exists?
            n155 = global read "Results_plotter_Global.vi" "Description"() -> (w511:string[])
            n156 = Empty String/Path?(string/path=w513) -> (empty?=w512:bool)
            n157 = case shown="False" w517 {
              tunnel: w523 -> [w530 _]
              tunnel: w511 -> [w529 _]
              tunnel: [w525 w536] -> w514
              tunnel: w522 -> [w528 w537]
              tunnel: [w527 w537] -> w516
              tunnel: w515 -> [w524 w536]
              frame False {
                n158 = for {
                  tunnel: w530 -> [w532] mode=indexing
                  tunnel: w528 -> [w535]
                  tunnel: [w534] -> w527 mode=indexing
                  tunnel: w529 -> [w533]
                  tunnel: [w531] -> w526 mode=indexing
                  n159 = Index Array(array=w535, index=w532) -> (element=w534:string)
                  n160 = Index Array(array=w533, index=w532) -> (element=w531:string)
                }
                n161 = Build Array (concatenate)(w526, w524) -> (w525:string[][])
              }
              frame True {
              }
            }
            n162 = case shown="False" w512 {
              tunnel: [w540 ""] -> w518
              tunnel: w513 -> [w538 _]
              frame False {
                n163 = Initialize Array("", 10 ("Dimension Size")) -> (w543:string[])
                n164 = call "Asterisk_header.vi"("Channel names"=w543) -> ("Header string"=w542:string)
                n165 = Concatenate Strings(w538, "\n", "#" ("Substring"), w542) -> (w540:string)
              }
              frame True {
              }
            }
            n166 = call "Write_Ch_data_file.vi"("Append last row only"=w519, "Header string"=w518, "exists?"=w521, "Channel Values"=w514, "Channel names"=w516, "Filename"=w520) -> ()  [unwired: 1 in, 5 out]
          }
        }
      }
    }
  }
  "Output filename Out" <- w11
